vi "Standard Error Behavior.vi"() -> ()   [LabVIEW 2017, in "Transparent Assertions.Tests.lvlib"]
uses:
  Transparent Assertions.Tests.lvlib
  <vilib>/Utility/error.llb/Error Cluster From Error Code.vi
  <vilib>/ErrorRing/Error Ring.xnode
  src/Transparent Assertions/Transparent Assertions.lvlib
panel:
  out "error out":errorcluster
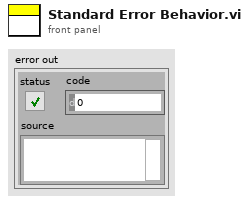
[diagram p1: front panel]
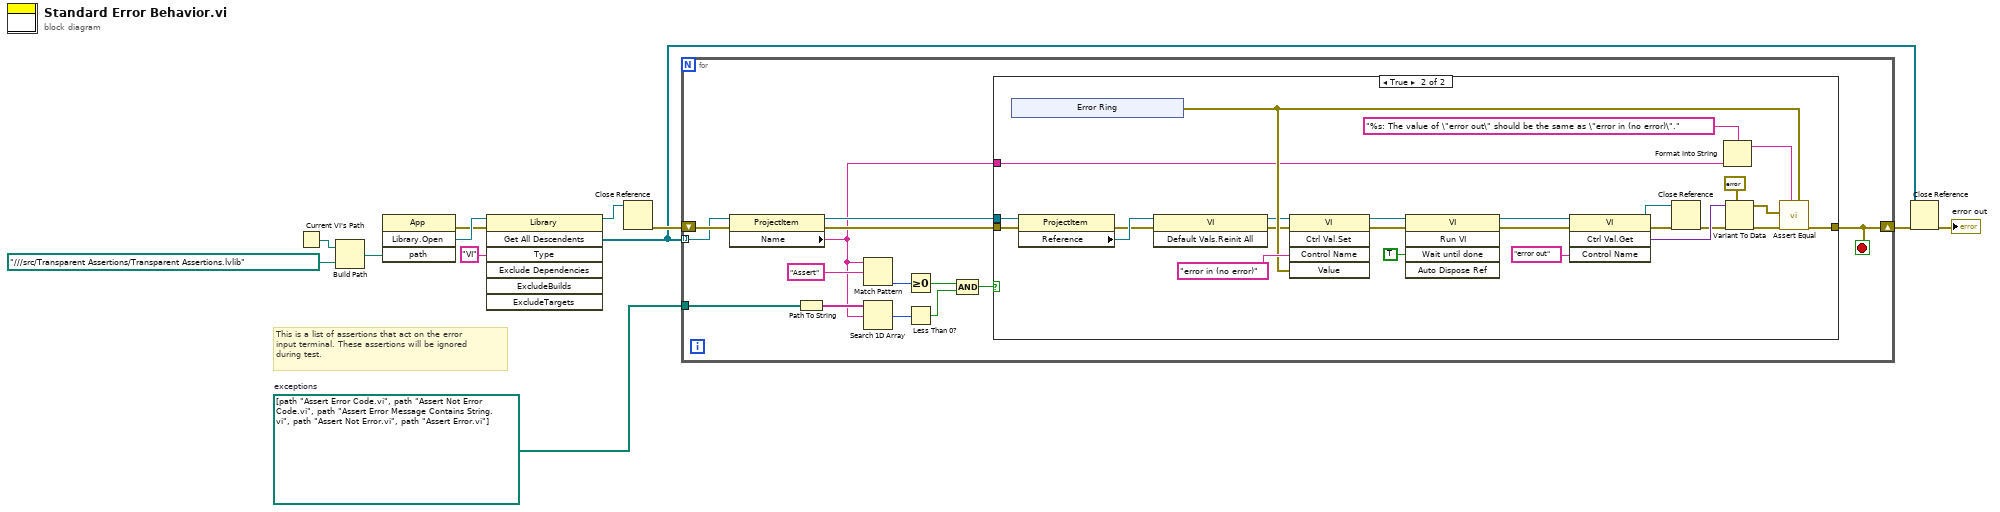
[diagram p0: block diagram]
diagram:
  w8 = path[] [path "Assert Error Code.vi", path "Assert Not Error Code.vi", path "Assert Error Message Contains String.vi", path "Assert Not Error.vi", path "Assert Error.vi"]  # exceptions
  # "This is a list of assertions that act on the error\ninput terminal. These assertions will be ignored\nduring test."
  n1 = Current VI's Path() -> (path=w11:path)
  n2 = Build Path(base path=w11, name or relative path=path "../../../src/Transparent Assertions/Transparent Assertions.lvlib") -> (appended path=w9:path)
  n3 = invoke class="App" method="Library.Open"("path"=w9) -> (error out=w2:errorcluster, "Open Library"=w5:refnum<vi>)  [unwired: 3 in, 2 out]
  n4 = invoke class="Library" method="Get All Descendents"(reference=w5, error in=w2, "Type"="VI") -> (reference out=w3:refnum<vi>, "All Descendents"=w1:refnum<vi>[])  [unwired: 4 in, 5 out]
  n5 = Close Reference(reference=w3) -> (error out=w6:errorcluster)  [unwired: 1 in]
  n6 = for {
    tunnel: w1 -> [w25] mode=indexing
    tunnel: w8 -> [w20]
    shift-right: [w21] -> w12
    shift-left: w6 -> [w26]
    stop <- w21 stop-if-true
    n7 = property class="ProjectItem"(reference=w25, error in=w26) -> (reference out=w23:refnum<vi>, error out=w22:errorcluster, "Name"=w13:string)
    n8 = Path To String(path=w20) -> (string=w19:string[])
    n9 = Match Pattern(string=w13, regular expression="Assert") -> (offset past match=w18:i32)  [unwired: 1 in, 3 out]
    n10 = Search 1D Array(1D array=w19, element=w13) -> (index of element=w16:i32)  [unwired: 1 in]
    n11 = Greater Or Equal To 0?(x=w18) -> (x >= 0?=w17:bool)
    n12 = Less Than 0?(x=w16) -> (x < 0?=w15:bool)
    n13 = Compound Arithmetic op=AND(w17, w15) -> (w14:bool)
    n14 = case shown="True" w14 {
      tunnel: w23 -> [_ w38]
      tunnel: w22 -> [w27 w37]
      tunnel: [w27 w44] -> w21
      tunnel: w13 -> [_ w29]
      frame False {
      }
      frame True {
        n15 = xnode "Error Ring"() -> ("error out"=w43:errorcluster)
        n16 = property class="ProjectItem"(reference=w38, error in=w37) -> (error out=w33:errorcluster, "Reference"=w34:refnum<vi>)  [unwired: 1 out]
        n17 = invoke class="VI" method="Default Vals.Reinit All"(reference=w34, error in=w33) -> (reference out=w35:refnum<vi>, error out=w36:errorcluster)  [unwired: 1 in, 1 out]
        n18 = invoke class="VI" method="Ctrl Val.Set"(reference=w35, error in=w36, "Control Name"="error in (no error)", "Value"=w43) -> (reference out=w50:refnum<vi>, error out=w51:errorcluster)  [unwired: 1 in, 3 out]
        n19 = invoke class="VI" method="Run VI"(reference=w50, error in=w51, "Wait until done"=TRUE ("Wait Until Done")) -> (reference out=w47:refnum<vi>, error out=w48:errorcluster)  [unwired: 2 in, 3 out]
        n20 = invoke class="VI" method="Ctrl Val.Get"(reference=w47, error in=w48, "Control Name"="error out") -> (reference out=w31:refnum<vi>, error out=w45:errorcluster, "Get Control Value Variant"=w41:variant)  [unwired: 1 in, 1 out]
        n21 = Close Reference(reference=w31, error in (no error)=w45) -> (error out=w32:errorcluster)
        n22 = Format Into String(format string="%s: The value of \"error out\" should be the same as \"error in (no error)\"." ("Message (\"\")"), w29) -> (resulting string=w28:string)  [unwired: 2 in, 1 out]
        n23 = Variant To Data(error in=w32, type=errorcluster {"status"=FALSE, "code"=0, "source"=""} ("error constant"), Variant=w41) -> (data=w39:errorcluster, error out=w42:errorcluster)
        n24 = call "Assert Equal.vi"("Expected"=w43, "Message (\"\")"=w28, "error in (no error)"=w42, "Actual"=w39) -> ("error out"=w44:errorcluster)  [unwired: 7 in]
      }
    }
  }
  n25 = Close Reference(reference=w1, error in (no error)=w12) -> (error out=→"error out":errorcluster)
